vi "诊断标定4.vi"(8 "CAN端口":u16(ring), 9 "设备索引号":u16(ring), 10 "CAN卡类型":u32(ring)=4) -> ()   [LabVIEW 2013] (continued)
            n2064 = property on="SOH(%)" class="DigNum (严格)"("Disabled"=w3261) -> ()  [unwired: 2 in, 2 out]
            n2065 = property on="电池额定容量(A)" class="DigNum (严格)"("Disabled"=w3261) -> ()  [unwired: 2 in, 2 out]
            n2066 = property on="SOC(%)" class="DigNum (严格)"("Disabled"=w3261) -> ()  [unwired: 2 in, 2 out]
            n2067 = local read "从板个数"() -> (w3259:dbl)
            n2068 = property on="系统时钟" class="Str"("Disabled"=w3261) -> ()  [unwired: 2 in, 2 out]
            n2069 = property on="配置文件版本" class="Str"("Disabled"=w3261) -> ()  [unwired: 2 in, 2 out]
            n2070 = property on="车架(牌)号" class="Str"("Disabled"=w3261) -> ()  [unwired: 2 in, 2 out]
            n2071 = property on="产品编号" class="Str"("Disabled"=w3261) -> ()  [unwired: 2 in, 2 out]
            n2072 = control-ref of="项目信息"() -> (w3260:refnum<vi>)
            n2073 = stacked-sequence {
              tunnel: w3260 -> [w3272 w3275]
              tunnel: w3259 -> [w3265 w3274]
              frame #0 {
                n2074 = Multiply(x=w3265, y=4.0) -> (x*y=w3267:dbl)
                n2075 = Compound Arithmetic op=ADD(24.0 ("值"), w3267) -> (w3269:dbl)
                n2076 = Bundle(w3269, 0) -> (w3271:cluster{dbl, i32})  [unwired: 1 out]
                n2077 = property class="Tbl (严格)"(reference=w3272, "Index Values"=w3271) -> ()  [unwired: 1 in, 2 out]
              }
              frame #1 {
                n2078 = for {
                  N: 20 -> [_]
                  tunnel: w3275 -> [w3285]
                  tunnel: w3274 -> [w3280]
                  i -> [w3279]
                  n2079 = Multiply(x=4.0, y=w3280) -> (x*y=w3277:dbl)
                  n2080 = Compound Arithmetic op=ADD(24.0 ("值"), w3277, w3279) -> (w3282:dbl)
                  n2081 = Bundle(w3282, 0) -> (w3284:cluster{dbl, i32})  [unwired: 1 out]
                  n2082 = property class="Tbl (严格)"(reference=w3285, "Active Cell"=w3284, "Cell BG Color"=u32 6618880) -> ()  [unwired: 1 in, 2 out]
                }
              }
            }
            n2083 = Select(t=1, s=w3252, f=0) -> (s? t:f=w3250:i32)
            n2084 = global read "功能码全局.vi" "主板项目信息4"() -> (w3257:bool[])
            n2085 = property on="项目信息" class="Tbl (严格)"("Disabled"=w3250) -> ()  [unwired: 2 in, 2 out]
            n2086 = Index Array(array=w3257, index #1=5 ("索引"), index #2=6 ("索引")) -> (element #1=w3255:bool, element #2=w3254:bool)
            n2087 = Not(x=w3263) -> (.not. x?=w3262:bool)
          }
          frame "SOC" {
            w3295 = 2
            w3297 = FALSE
            n2088 = property on="电池实际容量(A)" class="DigNum (严格)"("Disabled"=w3295) -> ()  [unwired: 2 in, 2 out]
            n2089 = property on="使用者" class="DigNum (严格)"("Disabled"=w3295) -> ()  [unwired: 2 in, 2 out]
            n2090 = property on="SOH(%)" class="DigNum (严格)"("Disabled"=w3295) -> ()  [unwired: 2 in, 2 out]
            n2091 = property on="电池额定容量(A)" class="DigNum (严格)"("Disabled"=w3295) -> ()  [unwired: 2 in, 2 out]
            n2092 = property on="系统时钟" class="Str"("Disabled"=w3295) -> ()  [unwired: 2 in, 2 out]
            n2093 = property on="配置文件版本" class="Str"("Disabled"=w3295) -> ()  [unwired: 2 in, 2 out]
            n2094 = property on="车架(牌)号" class="Str"("Disabled"=w3295) -> ()  [unwired: 2 in, 2 out]
            n2095 = property on="项目信息" class="Tbl (严格)"("Disabled"=w3295) -> ()  [unwired: 2 in, 2 out]
            n2096 = property on="产品编号" class="Str"("Disabled"=w3295) -> ()  [unwired: 2 in, 2 out]
            n2097 = Select(t=0, s=w3287, f=1) -> (s? t:f=w3286:i32)
            n2098 = property on="SOC(%)" class="DigNum (严格)"("Disabled"=w3286) -> ()  [unwired: 2 in, 2 out]
            n2099 = global read "功能码全局.vi" "主板项目信息7"() -> (w3293:bool[])
            n2100 = Index Array(array=w3293, index #1=2 ("索引"), index #2=5 ("索引")) -> (element #1=w3291:bool, element #2=w3290:bool)
            n2101 = Not(x=w3297) -> (.not. x?=w3296:bool)
          }
          frame "电池额定实际容量" {
            w3308 = 2
            w3310 = FALSE
            n2102 = property on="使用者" class="DigNum (严格)"("Disabled"=w3308) -> ()  [unwired: 2 in, 2 out]
            n2103 = property on="SOH(%)" class="DigNum (严格)"("Disabled"=w3308) -> ()  [unwired: 2 in, 2 out]
            n2104 = property on="SOC(%)" class="DigNum (严格)"("Disabled"=w3308) -> ()  [unwired: 2 in, 2 out]
            n2105 = property on="系统时钟" class="Str"("Disabled"=w3308) -> ()  [unwired: 2 in, 2 out]
            n2106 = property on="配置文件版本" class="Str"("Disabled"=w3308) -> ()  [unwired: 2 in, 2 out]
            n2107 = property on="车架(牌)号" class="Str"("Disabled"=w3308) -> ()  [unwired: 2 in, 2 out]
            n2108 = property on="项目信息" class="Tbl (严格)"("Disabled"=w3308) -> ()  [unwired: 2 in, 2 out]
            n2109 = property on="产品编号" class="Str"("Disabled"=w3308) -> ()  [unwired: 2 in, 2 out]
            n2110 = Select(t=0, s=w3300, f=1) -> (s? t:f=w3299:i32)
            n2111 = property on="电池实际容量(A)" class="DigNum (严格)"("Disabled"=w3299) -> ()  [unwired: 2 in, 2 out]
            n2112 = property on="电池额定容量(A)" class="DigNum (严格)"("Disabled"=w3299) -> ()  [unwired: 2 in, 2 out]
            n2113 = global read "功能码全局.vi" "主板项目信息7"() -> (w3306:bool[])
            n2114 = Index Array(array=w3306, index #1=3 ("索引"), index #2=6 ("索引")) -> (element #1=w3304:bool, element #2=w3303:bool)
            n2115 = Not(x=w3310) -> (.not. x?=w3309:bool)
          }
          frame "配置文件版本" {
            w3322 = 2
            w3324 = FALSE
            n2116 = property on="使用者" class="DigNum (严格)"("Disabled"=w3322) -> ()  [unwired: 2 in, 2 out]
            n2117 = property on="SOH(%)" class="DigNum (严格)"("Disabled"=w3322) -> ()  [unwired: 2 in, 2 out]
            n2118 = property on="SOC(%)" class="DigNum (严格)"("Disabled"=w3322) -> ()  [unwired: 2 in, 2 out]
            n2119 = property on="电池实际容量(A)" class="DigNum (严格)"("Disabled"=w3322) -> ()  [unwired: 2 in, 2 out]
            n2120 = property on="电池额定容量(A)" class="DigNum (严格)"("Disabled"=w3322) -> ()  [unwired: 2 in, 2 out]
            n2121 = property on="系统时钟" class="Str"("Disabled"=w3322) -> ()  [unwired: 2 in, 2 out]
            n2122 = property on="车架(牌)号" class="Str"("Disabled"=w3322) -> ()  [unwired: 2 in, 2 out]
            n2123 = property on="项目信息" class="Tbl (严格)"("Disabled"=w3322) -> ()  [unwired: 2 in, 2 out]
            n2124 = property on="产品编号" class="Str"("Disabled"=w3322) -> ()  [unwired: 2 in, 2 out]
            n2125 = Select(t=0, s=w3313, f=1) -> (s? t:f=w3312:i32)
            n2126 = property on="配置文件版本" class="Str"("Disabled"=w3312) -> ()  [unwired: 2 in, 2 out]
            n2127 = global read "功能码全局.vi" "主板项目信息5"() -> (w3320:bool[])
            n2128 = global read "功能码全局.vi" "主板项目信息6"() -> (w3319:bool[])
            n2129 = Index Array(array=w3320, index=6 ("索引")) -> (element=w3317:bool)
            n2130 = Index Array(array=w3319, index=7 ("索引")) -> (element=w3316:bool)
            n2131 = Not(x=w3324) -> (.not. x?=w3323:bool)
          }
          frame "参数修改记录" {
            w3336 = 2
            w3338 = FALSE
            n2132 = property on="SOH(%)" class="DigNum (严格)"("Disabled"=w3336) -> ()  [unwired: 2 in, 2 out]
            n2133 = property on="SOC(%)" class="DigNum (严格)"("Disabled"=w3336) -> ()  [unwired: 2 in, 2 out]
            n2134 = property on="电池实际容量(A)" class="DigNum (严格)"("Disabled"=w3336) -> ()  [unwired: 2 in, 2 out]
            n2135 = property on="电池额定容量(A)" class="DigNum (严格)"("Disabled"=w3336) -> ()  [unwired: 2 in, 2 out]
            n2136 = property on="系统时钟" class="Str"("Disabled"=w3336) -> ()  [unwired: 2 in, 2 out]
            n2137 = property on="车架(牌)号" class="Str"("Disabled"=w3336) -> ()  [unwired: 2 in, 2 out]
            n2138 = property on="配置文件版本" class="Str"("Disabled"=w3336) -> ()  [unwired: 2 in, 2 out]
            n2139 = property on="项目信息" class="Tbl (严格)"("Disabled"=w3336) -> ()  [unwired: 2 in, 2 out]
            n2140 = property on="产品编号" class="Str"("Disabled"=w3336) -> ()  [unwired: 2 in, 2 out]
            n2141 = Select(t=0, s=w3327, f=1) -> (s? t:f=w3326:i32)
            n2142 = property on="使用者" class="DigNum (严格)"("Disabled"=w3326) -> ()  [unwired: 2 in, 2 out]
            n2143 = global read "功能码全局.vi" "主板项目信息7"() -> (w3333:bool[])
            n2144 = global read "功能码全局.vi" "主板项目信息5"() -> (w3334:bool[])
            n2145 = Index Array(array=w3333, index=0 ("索引")) -> (element=w3331:bool)
            n2146 = Index Array(array=w3334, index=7 ("索引")) -> (element=w3330:bool)
            n2147 = Not(x=w3338) -> (.not. x?=w3337:bool)
          }
          frame "车牌号" {
            w3350 = 2
            w3352 = FALSE
            n2148 = property on="SOH(%)" class="DigNum (严格)"("Disabled"=w3350) -> ()  [unwired: 2 in, 2 out]
            n2149 = property on="使用者" class="DigNum (严格)"("Disabled"=w3350) -> ()  [unwired: 2 in, 2 out]
            n2150 = property on="SOC(%)" class="DigNum (严格)"("Disabled"=w3350) -> ()  [unwired: 2 in, 2 out]
            n2151 = property on="电池实际容量(A)" class="DigNum (严格)"("Disabled"=w3350) -> ()  [unwired: 2 in, 2 out]
            n2152 = property on="电池额定容量(A)" class="DigNum (严格)"("Disabled"=w3350) -> ()  [unwired: 2 in, 2 out]
            n2153 = property on="系统时钟" class="Str"("Disabled"=w3350) -> ()  [unwired: 2 in, 2 out]
            n2154 = property on="配置文件版本" class="Str"("Disabled"=w3350) -> ()  [unwired: 2 in, 2 out]
            n2155 = property on="项目信息" class="Tbl (严格)"("Disabled"=w3350) -> ()  [unwired: 2 in, 2 out]
            n2156 = property on="产品编号" class="Str"("Disabled"=w3350) -> ()  [unwired: 2 in, 2 out]
            n2157 = Select(t=0, s=w3341, f=1) -> (s? t:f=w3340:i32)
            n2158 = property on="车架(牌)号" class="Str"("Disabled"=w3340) -> ()  [unwired: 2 in, 2 out]
            n2159 = global read "功能码全局.vi" "主板项目信息7"() -> (w3347:bool[])
            n2160 = global read "功能码全局.vi" "主板项目信息6"() -> (w3348:bool[])
            n2161 = Index Array(array=w3347, index=1 ("索引")) -> (element=w3345:bool)
            n2162 = Index Array(array=w3348, index=0 ("索引")) -> (element=w3344:bool)
            n2163 = Not(x=w3352) -> (.not. x?=w3351:bool)
          }
          frame "SOH" {
            w3363 = 2
            w3365 = FALSE
            n2164 = property on="使用者" class="DigNum (严格)"("Disabled"=w3363) -> ()  [unwired: 2 in, 2 out]
            n2165 = property on="SOC(%)" class="DigNum (严格)"("Disabled"=w3363) -> ()  [unwired: 2 in, 2 out]
            n2166 = property on="电池实际容量(A)" class="DigNum (严格)"("Disabled"=w3363) -> ()  [unwired: 2 in, 2 out]
            n2167 = property on="电池额定容量(A)" class="DigNum (严格)"("Disabled"=w3363) -> ()  [unwired: 2 in, 2 out]
            n2168 = property on="系统时钟" class="Str"("Disabled"=w3363) -> ()  [unwired: 2 in, 2 out]
            n2169 = property on="配置文件版本" class="Str"("Disabled"=w3363) -> ()  [unwired: 2 in, 2 out]
            n2170 = property on="项目信息" class="Tbl (严格)"("Disabled"=w3363) -> ()  [unwired: 2 in, 2 out]
            n2171 = property on="产品编号" class="Str"("Disabled"=w3363) -> ()  [unwired: 2 in, 2 out]
            n2172 = property on="车架(牌)号" class="Str"("Disabled"=w3363) -> ()  [unwired: 2 in, 2 out]
            n2173 = Select(t=0, s=w3355, f=1) -> (s? t:f=w3354:i32)
            n2174 = property on="SOH(%)" class="DigNum (严格)"("Disabled"=w3354) -> ()  [unwired: 2 in, 2 out]
            n2175 = global read "功能码全局.vi" "主板项目信息7"() -> (w3362:bool[])
            n2176 = Index Array(array=w3362, index #1=4 ("索引"), index #2=7 ("索引")) -> (element #1=w3359:bool, element #2=w3358:bool)
            n2177 = Not(x=w3365) -> (.not. x?=w3364:bool)
          }
          frame "SOC过低(2)", "SOC过高(2)", "SOH过低(2)", "充电电流过高(2)", "单体电压过低(2)", "单体电压过高(2)", "单组电压不均衡(2)", "单组温度不均衡(2)", "二级故障阀值", "放电电流过高(2)", "极柱温度过高(2)", "内阻过大(2)", "温度过低(2)", "温度过高(2)", "整组电压不均衡(2)", "整组温度不均衡(2)", "总电压过低(2)", "总电压过高(2)" {
            w3376 = FALSE
            n2178 = Select(t=0, s=w3368, f=1) -> (s? t:f=w3367:i32)
            n2179 = property on="一级故障 2" class="Clust (严格)"("DisabledEnum"=w3367) -> ()  [unwired: 2 in, 2 out]
            n2180 = global read "功能码全局.vi" "主板故障阀值9"() -> (w3374:bool[])
            n2181 = Index Array(array=w3374, index #1=3 ("索引"), index #2=6 ("索引")) -> (element #1=w3372:bool, element #2=w3371:bool)
            n2182 = Not(x=w3376) -> (.not. x?=w3377:bool)
          }
          frame "SOC过低(3)", "SOC过高(3)", "SOH过低(3)", "充电电流过高(3)", "单体电压过低(3)", "单体电压过高(3)", "单组电压不均衡(3)", "单组温度不均衡(3)", "放电电流过高(3)", "极柱温度过高(3)", "内阻过大(3)", "三级故障阀值", "温度过低(3)", "温度过高(3)", "整组电压不均衡(3)", "整组温度不均衡(3)", "总电压过低(3)", "总电压过高(3)" {
            w3389 = FALSE
            n2183 = Select(t=0, s=w3380, f=1) -> (s? t:f=w3379:i32)
            n2184 = property on="一级故障 3" class="Clust (严格)"("DisabledEnum"=w3379) -> ()  [unwired: 2 in, 2 out]
            n2185 = global read "功能码全局.vi" "主板故障阀值9"() -> (w3386:bool[])
            n2186 = Index Array(array=w3386, index #1=4 ("索引"), index #2=7 ("索引")) -> (element #1=w3384:bool, element #2=w3383:bool)
            n2187 = Not(x=w3389) -> (.not. x?=w3388:bool)
          }
          frame "SOC过低", "SOC过高", "SOH过低", "充电电流过高", "单体电压过低", "单体电压过高", "单组电压不均衡", "单组温度不均衡", "放电电流过高", "极柱温度过高", "内阻过大", "温度过低", "温度过高", "一级故障阀值", "整组电压不均衡", "整组温度不均衡", "总电压过低", "总电压过高" {
            w3401 = FALSE
            n2188 = Select(t=0, s=w3392, f=1) -> (s? t:f=w3391:i32)
            n2189 = property on="一级故障" class="Clust (严格)"("DisabledEnum"=w3391) -> ()  [unwired: 2 in, 2 out]
            n2190 = global read "功能码全局.vi" "主板故障阀值9"() -> (w3398:bool[])
            n2191 = Index Array(array=w3398, index #1=2 ("索引"), index #2=5 ("索引")) -> (element #1=w3396:bool, element #2=w3395:bool)
            n2192 = Not(x=w3401) -> (.not. x?=w3400:bool)
          }
          frame "充电控制参数", "电流步长", "最大允许充电电流", "最大允许充电温度", "最大允许单体电压", "最大允许总电压", "最小允许充电电流", "最小允许充电温度", "最小允许单体电压" {
            w3403 = 2
            w3414 = FALSE
            n2193 = property on="风机开启温度" class="DigNum (严格)"("Disabled"=w3403) -> ()  [unwired: 2 in, 2 out]
            n2194 = property on="风机关闭温度" class="DigNum (严格)"("Disabled"=w3403) -> ()  [unwired: 2 in, 2 out]
            n2195 = property on="加热开启温度" class="DigNum (严格)"("Disabled"=w3403) -> ()  [unwired: 2 in, 2 out]
            n2196 = property on="加热关闭温度" class="DigNum (严格)"("Disabled"=w3403) -> ()  [unwired: 2 in, 2 out]
            n2197 = property on="风机开启温差" class="DigNum (严格)"("Disabled"=w3403) -> ()  [unwired: 2 in, 2 out]
            n2198 = property on="风机关闭温差" class="DigNum (严格)"("Disabled"=w3403) -> ()  [unwired: 2 in, 2 out]
            n2199 = property on="加热控制参数" class="Clust (严格)"("DisabledEnum"=w3403) -> ()  [unwired: 2 in, 2 out]
            n2200 = Select(t=0, s=w3405, f=1) -> (s? t:f=w3404:i32)
            n2201 = property on="最大允许总电压" class="DigNum (严格)"("Disabled"=w3404) -> ()  [unwired: 2 in, 2 out]
            n2202 = property on="最大允许充电温度" class="DigNum (严格)"("Disabled"=w3404) -> ()  [unwired: 2 in, 2 out]
            n2203 = property on="最小允许充电温度" class="DigNum (严格)"("Disabled"=w3404) -> ()  [unwired: 2 in, 2 out]
            n2204 = property on="电流步长" class="DigNum (严格)"("Disabled"=w3404) -> ()  [unwired: 2 in, 2 out]
            n2205 = property on="最大允许单体电压" class="DigNum (严格)"("Disabled"=w3404) -> ()  [unwired: 2 in, 2 out]
            n2206 = property on="最小允许单体电压" class="DigNum (严格)"("Disabled"=w3404) -> ()  [unwired: 2 in, 2 out]
            n2207 = property on="最大允许充电电流" class="DigNum (严格)"("Disabled"=w3404) -> ()  [unwired: 2 in, 2 out]
            n2208 = property on="最小允许充电电流" class="DigNum (严格)"("Disabled"=w3404) -> ()  [unwired: 2 in, 2 out]
            n2209 = global read "功能码全局.vi" "主板控制类信息10"() -> (w3411:bool[])
            n2210 = Index Array(array=w3411, index #1=5 ("索引"), index #2=7 ("索引")) -> (element #1=w3409:bool, element #2=w3408:bool)
            n2211 = Not(x=w3414) -> (.not. x?=w3413:bool)
          }
          frame "风机关闭温差", "风机关闭温度", "风机开启温差", "风机开启温度", "加热关闭温差", "加热关闭温度", "加热开启温度", "加热控制参数" {
            w3425 = 2
            w3427 = FALSE
            n2212 = Select(t=0, s=w3417, f=1) -> (s? t:f=w3416:i32)
            n2213 = property on="加热控制参数" class="Clust (严格)"("DisabledEnum"=w3416) -> ()  [unwired: 2 in, 2 out]
            n2214 = property on="风机开启温度" class="DigNum (严格)"("Disabled"=w3416) -> ()  [unwired: 2 in, 2 out]
            n2215 = property on="风机关闭温度" class="DigNum (严格)"("Disabled"=w3416) -> ()  [unwired: 2 in, 2 out]
            n2216 = property on="加热开启温度" class="DigNum (严格)"("Disabled"=w3416) -> ()  [unwired: 2 in, 2 out]
            n2217 = property on="加热关闭温度" class="DigNum (严格)"("Disabled"=w3416) -> ()  [unwired: 2 in, 2 out]
            n2218 = property on="风机开启温差" class="DigNum (严格)"("Disabled"=w3416) -> ()  [unwired: 2 in, 2 out]
            n2219 = property on="风机关闭温差" class="DigNum (严格)"("Disabled"=w3416) -> ()  [unwired: 2 in, 2 out]
            n2220 = property on="最大允许总电压" class="DigNum (严格)"("Disabled"=w3425) -> ()  [unwired: 2 in, 2 out]
            n2221 = property on="最大允许充电温度" class="DigNum (严格)"("Disabled"=w3425) -> ()  [unwired: 2 in, 2 out]
            n2222 = property on="最小允许充电温度" class="DigNum (严格)"("Disabled"=w3425) -> ()  [unwired: 2 in, 2 out]
            n2223 = property on="电流步长" class="DigNum (严格)"("Disabled"=w3425) -> ()  [unwired: 2 in, 2 out]
            n2224 = property on="最大允许单体电压" class="DigNum (严格)"("Disabled"=w3425) -> ()  [unwired: 2 in, 2 out]
            n2225 = property on="最小允许单体电压" class="DigNum (严格)"("Disabled"=w3425) -> ()  [unwired: 2 in, 2 out]
            n2226 = property on="最大允许充电电流" class="DigNum (严格)"("Disabled"=w3425) -> ()  [unwired: 2 in, 2 out]
            n2227 = property on="最小允许充电电流" class="DigNum (严格)"("Disabled"=w3425) -> ()  [unwired: 2 in, 2 out]
            n2228 = global read "功能码全局.vi" "主板控制类信息10"() -> (w3423:bool[])
            n2229 = Index Array(array=w3423, index #1=4 ("索引"), index #2=6 ("索引")) -> (element #1=w3421:bool, element #2=w3420:bool)
            n2230 = Not(x=w3427) -> (.not. x?=w3426:bool)
          }
          frame "电池信息" {
            w3439 = FALSE
            n2231 = Select(t=0, s=w3430, f=1) -> (s? t:f=w3429:i32)
            n2232 = property on="电池串联" class="DigNum (严格)"("Disabled"=w3429) -> ()  [unwired: 2 in, 2 out]
            n2233 = property on="电池并联" class="DigNum (严格)"("Disabled"=w3429) -> ()  [unwired: 2 in, 2 out]
            n2234 = property on="电池包额定容量" class="DigNum (严格)"("Disabled"=w3429) -> ()  [unwired: 2 in, 2 out]
            n2235 = property on="电池包额定能量" class="DigNum (严格)"("Disabled"=w3429) -> ()  [unwired: 2 in, 2 out]
            n2236 = property on="电池包额定总电压" class="DigNum (严格)"("Disabled"=w3429) -> ()  [unwired: 2 in, 2 out]
            n2237 = property on="实际容量" class="DigNum (严格)"("Disabled"=w3429) -> ()  [unwired: 2 in, 2 out]
            n2238 = property on="电池包组号" class="Str"("Disabled"=w3429) -> ()  [unwired: 2 in, 2 out]
            n2239 = property on="电池生产日期" class="Str"("Disabled"=w3429) -> ()  [unwired: 2 in, 2 out]
            n2240 = property on="电池厂家" class="Str"("Disabled"=w3429) -> ()  [unwired: 2 in, 2 out]
            n2241 = property on="电池类型" class="Str"("Disabled"=w3429) -> ()  [unwired: 2 in, 2 out]
            n2242 = property on="累计充电总安时" class="DigNum (严格)"("Disabled"=w3429) -> ()  [unwired: 2 in, 2 out]
            n2243 = property on="累计放电总安时" class="DigNum (严格)"("Disabled"=w3429) -> ()  [unwired: 2 in, 2 out]
            n2244 = property on="电池放空次数" class="DigNum (严格)"("Disabled"=w3429) -> ()  [unwired: 2 in, 2 out]
            n2245 = property on="电池充满次数" class="DigNum (严格)"("Disabled"=w3429) -> ()  [unwired: 2 in, 2 out]
            n2246 = property on="电池充电次数" class="DigNum (严格)"("Disabled"=w3429) -> ()  [unwired: 2 in, 2 out]
            n2247 = global read "功能码全局.vi" "主板版本号11"() -> (w3436:bool[])
            n2248 = Index Array(array=w3436, index #1=0 ("索引"), index #2=1 ("索引")) -> (element #1=w3434:bool, element #2=w3433:bool)
            n2249 = Not(x=w3439) -> (.not. x?=w3438:bool)
          }
          frame "电池信息1" {
            w3450 = 2
            w3452 = FALSE
            n2250 = Select(t=0, s=w3441, f=1) -> (s? t:f=w3442:i32)
            n2251 = property on="电池生产日期" class="Str"("Disabled"=w3442) -> ()  [unwired: 2 in, 2 out]
            n2252 = property on="电池厂家" class="Str"("Disabled"=w3442) -> ()  [unwired: 2 in, 2 out]
            n2253 = property on="电池类型" class="Str"("Disabled"=w3442) -> ()  [unwired: 2 in, 2 out]
            n2254 = property on="电池串联" class="DigNum (严格)"("Disabled"=w3442) -> ()  [unwired: 2 in, 2 out]
            n2255 = property on="电池并联" class="DigNum (严格)"("Disabled"=w3442) -> ()  [unwired: 2 in, 2 out]
            n2256 = property on="电池包额定容量" class="DigNum (严格)"("Disabled"=w3442) -> ()  [unwired: 2 in, 2 out]
            n2257 = property on="电池包额定能量" class="DigNum (严格)"("Disabled"=w3442) -> ()  [unwired: 2 in, 2 out]
            n2258 = property on="电池包额定总电压" class="DigNum (严格)"("Disabled"=w3442) -> ()  [unwired: 2 in, 2 out]
            n2259 = property on="实际容量" class="DigNum (严格)"("Disabled"=w3442) -> ()  [unwired: 2 in, 2 out]
            n2260 = property on="累计充电总安时" class="DigNum (严格)"("Disabled"=w3450) -> ()  [unwired: 2 in, 2 out]
            n2261 = property on="累计放电总安时" class="DigNum (严格)"("Disabled"=w3450) -> ()  [unwired: 2 in, 2 out]
            n2262 = property on="电池放空次数" class="DigNum (严格)"("Disabled"=w3450) -> ()  [unwired: 2 in, 2 out]
            n2263 = property on="电池充满次数" class="DigNum (严格)"("Disabled"=w3450) -> ()  [unwired: 2 in, 2 out]
            n2264 = property on="电池充电次数" class="DigNum (严格)"("Disabled"=w3450) -> ()  [unwired: 2 in, 2 out]
            n2265 = property on="电池包组号" class="Str"("Disabled"=w3450) -> ()  [unwired: 2 in, 2 out]
            n2266 = global read "功能码全局.vi" "主板版本号11"() -> (w3448:bool[])
            n2267 = Index Array(array=w3448, index #1=0 ("索引"), index #2=1 ("索引")) -> (element #1=w3446:bool, element #2=w3445:bool)
            n2268 = Not(x=w3452) -> (.not. x?=w3451:bool)
          }
          frame "电池包组号" {
            w3463 = 2
            w3465 = FALSE
            n2269 = property on="电池生产日期" class="Str"("Disabled"=w3463) -> ()  [unwired: 2 in, 2 out]
            n2270 = property on="电池厂家" class="Str"("Disabled"=w3463) -> ()  [unwired: 2 in, 2 out]
            n2271 = property on="电池类型" class="Str"("Disabled"=w3463) -> ()  [unwired: 2 in, 2 out]
            n2272 = property on="电池串联" class="DigNum (严格)"("Disabled"=w3463) -> ()  [unwired: 2 in, 2 out]
            n2273 = property on="电池并联" class="DigNum (严格)"("Disabled"=w3463) -> ()  [unwired: 2 in, 2 out]
            n2274 = property on="电池包额定容量" class="DigNum (严格)"("Disabled"=w3463) -> ()  [unwired: 2 in, 2 out]
            n2275 = property on="电池包额定能量" class="DigNum (严格)"("Disabled"=w3463) -> ()  [unwired: 2 in, 2 out]
            n2276 = property on="电池包额定总电压" class="DigNum (严格)"("Disabled"=w3463) -> ()  [unwired: 2 in, 2 out]
            n2277 = property on="实际容量" class="DigNum (严格)"("Disabled"=w3463) -> ()  [unwired: 2 in, 2 out]
            n2278 = property on="累计充电总安时" class="DigNum (严格)"("Disabled"=w3463) -> ()  [unwired: 2 in, 2 out]
            n2279 = property on="累计放电总安时" class="DigNum (严格)"("Disabled"=w3463) -> ()  [unwired: 2 in, 2 out]
            n2280 = property on="电池放空次数" class="DigNum (严格)"("Disabled"=w3463) -> ()  [unwired: 2 in, 2 out]
            n2281 = property on="电池充满次数" class="DigNum (严格)"("Disabled"=w3463) -> ()  [unwired: 2 in, 2 out]
            n2282 = property on="电池充电次数" class="DigNum (严格)"("Disabled"=w3463) -> ()  [unwired: 2 in, 2 out]
            n2283 = Select(t=0, s=w3455, f=1) -> (s? t:f=w3454:i32)
            n2284 = property on="电池包组号" class="Str"("Disabled"=w3454) -> ()  [unwired: 2 in, 2 out]
            n2285 = global read "功能码全局.vi" "主板版本号11"() -> (w3461:bool[])
            n2286 = Index Array(array=w3461, index #1=0 ("索引"), index #2=1 ("索引")) -> (element #1=w3459:bool, element #2=w3458:bool)
            n2287 = Not(x=w3465) -> (.not. x?=w3464:bool)
          }
          frame "充放电安时" {
            w3476 = 2
            w3478 = FALSE
            n2288 = property on="电池生产日期" class="Str"("Disabled"=w3476) -> ()  [unwired: 2 in, 2 out]
            n2289 = property on="电池厂家" class="Str"("Disabled"=w3476) -> ()  [unwired: 2 in, 2 out]
            n2290 = property on="电池类型" class="Str"("Disabled"=w3476) -> ()  [unwired: 2 in, 2 out]
            n2291 = property on="电池串联" class="DigNum (严格)"("Disabled"=w3476) -> ()  [unwired: 2 in, 2 out]
            n2292 = property on="电池并联" class="DigNum (严格)"("Disabled"=w3476) -> ()  [unwired: 2 in, 2 out]
            n2293 = property on="电池包额定容量" class="DigNum (严格)"("Disabled"=w3476) -> ()  [unwired: 2 in, 2 out]
            n2294 = property on="电池包额定能量" class="DigNum (严格)"("Disabled"=w3476) -> ()  [unwired: 2 in, 2 out]
            n2295 = property on="电池包额定总电压" class="DigNum (严格)"("Disabled"=w3476) -> ()  [unwired: 2 in, 2 out]
            n2296 = property on="实际容量" class="DigNum (严格)"("Disabled"=w3476) -> ()  [unwired: 2 in, 2 out]
            n2297 = property on="电池放空次数" class="DigNum (严格)"("Disabled"=w3476) -> ()  [unwired: 2 in, 2 out]
            n2298 = property on="电池充满次数" class="DigNum (严格)"("Disabled"=w3476) -> ()  [unwired: 2 in, 2 out]
            n2299 = property on="电池充电次数" class="DigNum (严格)"("Disabled"=w3476) -> ()  [unwired: 2 in, 2 out]
            n2300 = Select(t=0, s=w3468, f=1) -> (s? t:f=w3467:i32)
            n2301 = property on="电池包组号" class="Str"("Disabled"=w3476) -> ()  [unwired: 2 in, 2 out]
            n2302 = property on="累计充电总安时" class="DigNum (严格)"("Disabled"=w3467) -> ()  [unwired: 2 in, 2 out]
            n2303 = property on="累计放电总安时" class="DigNum (严格)"("Disabled"=w3467) -> ()  [unwired: 2 in, 2 out]
            n2304 = global read "功能码全局.vi" "主板版本号11"() -> (w3474:bool[])
            n2305 = Index Array(array=w3474, index #1=0 ("索引"), index #2=1 ("索引")) -> (element #1=w3472:bool, element #2=w3471:bool)
            n2306 = Not(x=w3478) -> (.not. x?=w3477:bool)
          }
          frame "电池充放电次数" {
            w3489 = 2
            w3491 = FALSE
            n2307 = property on="电池生产日期" class="Str"("Disabled"=w3489) -> ()  [unwired: 2 in, 2 out]
            n2308 = property on="电池厂家" class="Str"("Disabled"=w3489) -> ()  [unwired: 2 in, 2 out]
            n2309 = property on="电池类型" class="Str"("Disabled"=w3489) -> ()  [unwired: 2 in, 2 out]
            n2310 = property on="电池串联" class="DigNum (严格)"("Disabled"=w3489) -> ()  [unwired: 2 in, 2 out]
            n2311 = property on="电池并联" class="DigNum (严格)"("Disabled"=w3489) -> ()  [unwired: 2 in, 2 out]
            n2312 = property on="电池包额定容量" class="DigNum (严格)"("Disabled"=w3489) -> ()  [unwired: 2 in, 2 out]
            n2313 = property on="电池包额定能量" class="DigNum (严格)"("Disabled"=w3489) -> ()  [unwired: 2 in, 2 out]
            n2314 = property on="电池包额定总电压" class="DigNum (严格)"("Disabled"=w3489) -> ()  [unwired: 2 in, 2 out]
            n2315 = property on="实际容量" class="DigNum (严格)"("Disabled"=w3489) -> ()  [unwired: 2 in, 2 out]
            n2316 = Select(t=0, s=w3481, f=1) -> (s? t:f=w3480:i32)
            n2317 = property on="电池放空次数" class="DigNum (严格)"("Disabled"=w3480) -> ()  [unwired: 2 in, 2 out]
            n2318 = property on="电池充满次数" class="DigNum (严格)"("Disabled"=w3480) -> ()  [unwired: 2 in, 2 out]
            n2319 = property on="电池充电次数" class="DigNum (严格)"("Disabled"=w3480) -> ()  [unwired: 2 in, 2 out]
            n2320 = property on="累计充电总安时" class="DigNum (严格)"("Disabled"=w3489) -> ()  [unwired: 2 in, 2 out]
            n2321 = property on="累计放电总安时" class="DigNum (严格)"("Disabled"=w3489) -> ()  [unwired: 2 in, 2 out]
            n2322 = property on="电池包组号" class="Str"("Disabled"=w3489) -> ()  [unwired: 2 in, 2 out]
            n2323 = global read "功能码全局.vi" "主板版本号11"() -> (w3487:bool[])
            n2324 = Index Array(array=w3487, index #1=0 ("索引"), index #2=1 ("索引")) -> (element #1=w3485:bool, element #2=w3484:bool)
            n2325 = Not(x=w3491) -> (.not. x?=w3490:bool)
          }
          frame "假", Default {
            w3496 = FALSE
            n2326 = Not(x=w3496) -> (.not. x?=w3495:bool)
          }
        }
        n2327 = property on="单个读取" class="Bool (严格)"("Visible"=w2991) -> ()  [unwired: 2 in, 2 out]
        n2328 = property on="单个写入" class="Bool (严格)"("Visible"=w2990) -> ()  [unwired: 2 in, 2 out]
        n2329 = local write "1"(w2998) -> ()
        n2330 = local write "1 2"(w2997) -> ()
        n2331 = local write "1 3"(w2996) -> ()
        n2332 = local write "1 4"(w2995) -> ()
        n2333 = local write "1 5"(w2994) -> ()
        n2334 = local write "1 11"(w2993) -> ()
        n2335 = local write "主板2"(w2999) -> ()
      }
      event "从板选项": Mouse Down {
        n2336 = event-data() -> ("CtlRef"=w3507:refnum<vi>)  [unwired: 8 out]
        n2337 = property class="Tree (严格)"(reference=w3507) -> ("Value"=w3506:string)  [unwired: 1 in, 2 out]
        n2338 = case shown="\"SOC过低(3)\", \"电压不均衡(3)\", \"电压过低(3)\", \"电压过高(3)\", \"三级故障阀值\", \"温度不均衡(3)\", \"温度过低(3)\", \"温度过高(3)\"" w3506 {
          tunnel: [T13."从板信息" ("等级 2") T13."从板信息" ("等级 2") T13."从板信息" ("等级 2") T13."从板信息" ("等级 2") T13."从板信息" ("等级 2") T13."从板信息" ("等级 2") T13."从板信息" ("等级 2") T13."一级故障阀值" ("等级 2") T13."二级故障阀值" ("等级 2") T13."三级故障阀值" ("等级 2") T13."快换参数" ("等级 2") T13."快换参数" ("等级 2") T13."快换参数" ("等级 2") T13."快换参数" ("等级 2") T13."快换参数" ("等级 2") T13."快换参数" ("等级 2") T13."快换参数" ("等级 2") T13."快换参数" ("等级 2") T13."从板信息" ("等级 2")] -> w3505
          tunnel: [w3516 w3521 w3531 w3542 w3573 w3606 w3630 w3661 w3669 w3677 w3682 w3691 w3700 w3710 w3720 w3731 w3742 w3752 w3754] -> w3504
          tunnel: [w3517 w3522 w3532 w3543 w3574 w3607 w3631 w3660 w3669 w3677 w3682 w3691 w3700 w3710 w3720 w3731 w3742 w3752 w3755] -> w3503
          tunnel: [w3517 w3522 w3532 w3543 w3574 w3607 w3631 w3661 w3668 w3677 w3682 w3691 w3700 w3710 w3720 w3731 w3742 w3752 w3755] -> w3502
          tunnel: [w3517 w3522 w3532 w3543 w3574 w3607 w3631 w3661 w3669 w3676 w3682 w3691 w3700 w3710 w3720 w3731 w3742 w3752 w3755] -> w3501
          tunnel: [w3517 w3522 w3532 w3543 w3574 w3607 w3631 w3661 w3669 w3677 w3681 w3690 w3699 w3709 w3719 w3730 w3741 w3751 w3755] -> w3500
          tunnel: [w3513 w3519 w3525 w3535 w3566 w3599 w3623 w3656 w3664 w3672 FALSE _ _ _ _ _ _ _ _] -> w3499
          tunnel: [w3510 w3519 w3524 w3534 w3565 w3598 w3622 w3655 w3663 w3671 _ _ _ _ _ _ _ _ _] -> w3498
          frame "从板号" {
            w3515 = 2
            w3517 = FALSE ("1 6")
            n2339 = property on="项目信息 2" class="Tbl (严格)"("Disabled"=w3515) -> ()  [unwired: 2 in, 2 out]
            n2340 = property on="加热控制参数" class="Clust (严格)"("Disabled"=w3515) -> ()  [unwired: 2 in, 2 out]
            n2341 = global read "功能码全局.vi" "16"() -> (w3512:bool[])
            n2342 = Index Array(array=w3512, index #1=4 ("索引"), index #2=6 ("索引")) -> (element #1=w3513:bool, element #2=w3510:bool)
            n2343 = Not(x=w3517) -> (.not. x?=w3516:bool)
          }
          frame "从板信息" {
            w3519 = TRUE
            w3520 = 0
            w3522 = FALSE ("1 6")
            n2344 = property on="项目信息 2" class="Tbl (严格)"("Disabled"=w3520) -> ()  [unwired: 2 in, 2 out]
            n2345 = property on="加热控制参数" class="Clust (严格)"("Disabled"=w3520) -> ()  [unwired: 2 in, 2 out]
            n2346 = Not(x=w3522) -> (.not. x?=w3521:bool)
          }
          frame "风机关闭温差", "风机关闭温度", "风机开启温差", "风机开启温度", "加热关闭温差", "加热关闭温度", "加热开启温度", "加热控制参数" {
            w3532 = FALSE ("1 6")
            n2347 = property on="项目信息 2" class="Tbl (严格)"("Disabled"=2) -> ()  [unwired: 2 in, 2 out]
            n2348 = property on="加热控制参数" class="Clust (严格)"("Disabled"=0) -> ()  [unwired: 2 in, 2 out]
            n2349 = global read "功能码全局.vi" "16"() -> (w3527:bool[])
            n2350 = Index Array(array=w3527, index #1=5 ("索引"), index #2=7 ("索引")) -> (element #1=w3525:bool, element #2=w3524:bool)
            n2351 = Not(x=w3532) -> (.not. x?=w3531:bool)
          }
          frame "电压起始值" {
            w3543 = FALSE ("1 6")
            n2352 = property on="项目信息 2" class="Tbl (严格)"("Disabled"=0) -> ()  [unwired: 2 in, 2 out]
            n2353 = property on="加热控制参数" class="Clust (严格)"("Disabled"=2) -> ()  [unwired: 2 in, 2 out]
            n2354 = control-ref of="项目信息 2"() -> (w3539:refnum<vi>)
            n2355 = stacked-sequence {
              tunnel: w3539 -> [w3548 w3550 w3559]
              frame #0 {
                n2356 = Bundle(0, 0) -> (w3547:cluster{i32, i32})  [unwired: 1 out]
                n2357 = property class="Tbl (严格)"(reference=w3548, "Index Values"=w3547) -> ()  [unwired: 1 in, 2 out]
              }
              frame #1 {
                n2358 = for {
                  N: 8 -> [_]
                  tunnel: w3550 -> [w3557]
                  i -> [w3552]
                  n2359 = Compound Arithmetic op=ADD(2 ("值"), w3552) -> (w3554:i32)
                  n2360 = Bundle(w3554, 0) -> (w3556:cluster{i32, i32})  [unwired: 1 out]
                  n2361 = property class="Tbl (严格)"(reference=w3557, "Active Cell"=w3556, "Cell BG Color"=u32 16448250) -> ()  [unwired: 1 in, 2 out]
                }
              }
              frame #2 {
                n2362 = for {
                  N: 2 -> [_]
                  tunnel: w3559 -> [w3564]
                  i -> [w3560]
                  n2363 = Bundle(w3560, 0) -> (w3563:cluster{i32, i32})  [unwired: 1 out]
                  n2364 = property class="Tbl (严格)"(reference=w3564, "Active Cell"=w3563, "Cell BG Color"=u32 6618880) -> ()  [unwired: 1 in, 2 out]
                }
              }
            }
            n2365 = global read "功能码全局.vi" "15"() -> (w3537:bool[])
            n2366 = Index Array(array=w3537, index #1=0 ("索引"), index #2=4 ("索引")) -> (element #1=w3535:bool, element #2=w3534:bool)
            n2367 = Not(x=w3543) -> (.not. x?=w3542:bool)
          }
          frame "通道电压节数" {
            w3574 = FALSE ("1 6")
            n2368 = property on="项目信息 2" class="Tbl (严格)"("Disabled"=0) -> ()  [unwired: 2 in, 2 out]
            n2369 = property on="加热控制参数" class="Clust (严格)"("Disabled"=2) -> ()  [unwired: 2 in, 2 out]
            n2370 = control-ref of="项目信息 2"() -> (w3570:refnum<vi>)
            n2371 = stacked-sequence {
              tunnel: w3570 -> [w3579 w3581 w3590]
              frame #0 {
                n2372 = Bundle(2, 0) -> (w3578:cluster{i32, i32})  [unwired: 1 out]
                n2373 = property class="Tbl (严格)"(reference=w3579, "Index Values"=w3578) -> ()  [unwired: 1 in, 2 out]
              }
              frame #1 {
                n2374 = for {
                  N: 8 -> [_]
                  tunnel: w3581 -> [w3588]
                  i -> [w3583]
                  n2375 = Compound Arithmetic op=ADD(12 ("值"), w3583) -> (w3585:i32)
                  n2376 = Bundle(w3585, 0) -> (w3587:cluster{i32, i32})  [unwired: 1 out]
                  n2377 = property class="Tbl (严格)"(reference=w3588, "Active Cell"=w3587, "Cell BG Color"=u32 16448250) -> ()  [unwired: 1 in, 2 out]
                }
              }
              frame #2 {
                n2378 = for {
                  N: 20 -> [_]
                  tunnel: w3590 -> [w3597]
                  i -> [w3593]
                  n2379 = Add(x=2, y=w3593) -> (x+y=w3592:i32)
                  n2380 = Bundle(w3592, 0) -> (w3596:cluster{i32, i32})  [unwired: 1 out]
                  n2381 = property class="Tbl (严格)"(reference=w3597, "Active Cell"=w3596, "Cell BG Color"=u32 6618880) -> ()  [unwired: 1 in, 2 out]
                }
              }
            }
            n2382 = global read "功能码全局.vi" "15"() -> (w3568:bool[])
            n2383 = Index Array(array=w3568, index #1=1 ("索引"), index #2=5 ("索引")) -> (element #1=w3566:bool, element #2=w3565:bool)
            n2384 = Not(x=w3574) -> (.not. x?=w3573:bool)
          }
          frame "保险位置" {
            w3607 = FALSE ("1 6")
            n2385 = property on="项目信息 2" class="Tbl (严格)"("Disabled"=0) -> ()  [unwired: 2 in, 2 out]
            n2386 = property on="加热控制参数" class="Clust (严格)"("Disabled"=2) -> ()  [unwired: 2 in, 2 out]
            n2387 = control-ref of="项目信息 2"() -> (w3603:refnum<vi>)
            n2388 = stacked-sequence {
              tunnel: w3603 -> [w3612 w3614]
              frame #0 {
                n2389 = Bundle(24, 0) -> (w3611:cluster{i32, i32})  [unwired: 1 out]
                n2390 = property class="Tbl (严格)"(reference=w3612, "Index Values"=w3611) -> ()  [unwired: 1 in, 2 out]
              }
              frame #1 {
                n2391 = for {
                  N: 20 -> [_]
                  tunnel: w3614 -> [w3621]
                  i -> [w3617]
                  n2392 = Add(x=24, y=w3617) -> (x+y=w3616:i32)
                  n2393 = Bundle(w3616, 0) -> (w3620:cluster{i32, i32})  [unwired: 1 out]
                  n2394 = property class="Tbl (严格)"(reference=w3621, "Active Cell"=w3620, "Cell BG Color"=u32 6618880) -> ()  [unwired: 1 in, 2 out]
                }
              }
            }
            n2395 = global read "功能码全局.vi" "15"() -> (w3601:bool[])
            n2396 = Index Array(array=w3601, index #1=2 ("索引"), index #2=6 ("索引")) -> (element #1=w3599:bool, element #2=w3598:bool)
            n2397 = Not(x=w3607) -> (.not. x?=w3606:bool)
          }
          frame "温度起始值" {
            w3631 = FALSE ("1 6")
            n2398 = property on="项目信息 2" class="Tbl (严格)"("Disabled"=0) -> ()  [unwired: 2 in, 2 out]
            n2399 = property on="加热控制参数" class="Clust (严格)"("Disabled"=2) -> ()  [unwired: 2 in, 2 out]
            n2400 = control-ref of="项目信息 2"() -> (w3627:refnum<vi>)
            n2401 = stacked-sequence {
              tunnel: w3627 -> [w3636 w3637 w3647]
              frame #0 {
                n2402 = Bundle(22, 0) -> (w3635:cluster{i32, i32})  [unwired: 1 out]
                n2403 = property class="Tbl (严格)"(reference=w3636, "Index Values"=w3635) -> ()  [unwired: 1 in, 2 out]
              }
              frame #1 {
                n2404 = for {
                  N: 10 -> [_]
                  tunnel: w3637 -> [w3645]
                  i -> [w3640]
                  n2405 = Compound Arithmetic op=ADD(24 ("值"), w3640) -> (w3642:i32)
                  n2406 = Bundle(w3642, 0) -> (w3644:cluster{i32, i32})  [unwired: 1 out]
                  n2407 = property class="Tbl (严格)"(reference=w3645, "Active Cell"=w3644, "Cell BG Color"=u32 16448250) -> ()  [unwired: 1 in, 2 out]
                }
              }
              frame #2 {
                n2408 = for {
                  N: 2 -> [_]
                  tunnel: w3647 -> [w3654]
                  i -> [w3650]
                  n2409 = Add(x=22, y=w3650) -> (x+y=w3649:i32)
                  n2410 = Bundle(w3649, 0) -> (w3653:cluster{i32, i32})  [unwired: 1 out]
                  n2411 = property class="Tbl (严格)"(reference=w3654, "Active Cell"=w3653, "Cell BG Color"=u32 6618880) -> ()  [unwired: 1 in, 2 out]
                }
              }
            }
            n2412 = global read "功能码全局.vi" "15"() -> (w3625:bool[])
            n2413 = Index Array(array=w3625, index #1=3 ("索引"), index #2=7 ("索引")) -> (element #1=w3623:bool, element #2=w3622:bool)
            n2414 = Not(x=w3631) -> (.not. x?=w3630:bool)
          }
          frame "SOC过低", "电压不均衡", "电压过低", "电压过高", "温度不均衡", "温度过低", "温度过高", "一级故障阀值" {
            w3661 = FALSE ("1 6")
            n2415 = global read "功能码全局.vi" "18"() -> (w3658:bool[])
            n2416 = Index Array(array=w3658, index #1=2 ("索引"), index #2=5 ("索引")) -> (element #1=w3656:bool, element #2=w3655:bool)
            n2417 = Not(x=w3661) -> (.not. x?=w3660:bool)
          }
          frame "SOC过低(2)", "电压不均衡(2)", "电压过低(2)", "电压过高(2)", "二级故障阀值", "温度不均衡(2)", "温度过低(2)", "温度过高(2)" {
            w3669 = FALSE ("1 6")
            n2418 = global read "功能码全局.vi" "18"() -> (w3666:bool[])
            n2419 = Index Array(array=w3666, index #1=3 ("索引"), index #2=6 ("索引")) -> (element #1=w3664:bool, element #2=w3663:bool)
            n2420 = Not(x=w3669) -> (.not. x?=w3668:bool)
          }
          frame "SOC过低(3)", "电压不均衡(3)", "电压过低(3)", "电压过高(3)", "三级故障阀值", "温度不均衡(3)", "温度过低(3)", "温度过高(3)" {
            w3677 = FALSE ("1 6")
            n2421 = global read "功能码全局.vi" "18"() -> (w3674:bool[])
            n2422 = Index Array(array=w3674, index #1=4 ("索引"), index #2=7 ("索引")) -> (element #1=w3672:bool, element #2=w3671:bool)
            n2423 = Not(x=w3677) -> (.not. x?=w3676:bool)
          }
          frame "快换参数" {
            w3682 = FALSE ("1 6")
            n2424 = property on="电池组信息" class="Clust (严格)"("Disabled"=0) -> ()  [unwired: 2 in, 2 out]
            n2425 = Not(x=w3682) -> (.not. x?=w3681:bool)
          }
          frame "电池包信息1" {
            w3684 = 2
            w3686 = 2
            w3688 = 0
            w3691 = FALSE ("1 6")
            n2426 = property on="电池类型" class="DigNum (严格)"("Disabled"=w3688) -> ()  [unwired: 2 in, 2 out]
            n2427 = property on="电池厂家" class="DigNum (严格)"("Disabled"=w3688) -> ()  [unwired: 2 in, 2 out]
            n2428 = property on="电池地区" class="DigNum (严格)"("Disabled"=w3688) -> ()  [unwired: 2 in, 2 out]
            n2429 = property on="电池组序号" class="DigNum (严格)"("Disabled"=w3688) -> ()  [unwired: 2 in, 2 out]
            n2430 = property on="电池包串联数" class="DigNum (严格)"("Disabled"=w3688) -> ()  [unwired: 2 in, 2 out]
            n2431 = property on="电池包并联数" class="DigNum (严格)"("Disabled"=w3688) -> ()  [unwired: 2 in, 2 out]
            n2432 = property on="电池包安时数" class="DigNum (严格)"("Disabled"=w3688) -> ()  [unwired: 2 in, 2 out]
            n2433 = property on="电池组信息" class="Clust (严格)"("Disabled"=0) -> ()  [unwired: 2 in, 2 out]
            n2434 = property on="车牌号" class="Str"("Disabled"=2) -> ()  [unwired: 2 in, 2 out]
            n2435 = property on="电池包序号" class="DigNum (严格)"("Disabled"=2) -> ()  [unwired: 2 in, 2 out]
            n2436 = property on="充电次数" class="DigNum (严格)"("Disabled"=w3686) -> ()  [unwired: 2 in, 2 out]
            n2437 = property on="充满电时间" class="DigNum (严格)"("Disabled"=w3686) -> ()  [unwired: 2 in, 2 out]
            n2438 = property on="放空时间" class="DigNum (严格)"("Disabled"=w3686) -> ()  [unwired: 2 in, 2 out]
            n2439 = property on="最大允许单体电压" class="DigNum (严格)"("Disabled"=w3684) -> ()  [unwired: 2 in, 2 out]
            n2440 = property on="最大允许总电压" class="DigNum (严格)"("Disabled"=w3684) -> ()  [unwired: 2 in, 2 out]
            n2441 = property on="最大允许温度" class="DigNum (严格)"("Disabled"=w3684) -> ()  [unwired: 2 in, 2 out]
            n2442 = property on="最小允许温度" class="DigNum (严格)"("Disabled"=w3684) -> ()  [unwired: 2 in, 2 out]
            n2443 = property on="最大允许充电电流" class="DigNum (严格)"("Disabled"=w3684) -> ()  [unwired: 2 in, 2 out]
            n2444 = property on="最小允许充电电流" class="DigNum (严格)"("Disabled"=w3684) -> ()  [unwired: 2 in, 2 out]
            n2445 = property on="最小允许单体电压" class="DigNum (严格)"("Disabled"=w3684) -> ()  [unwired: 2 in, 2 out]
            n2446 = property on="电流步长" class="DigNum (严格)"("Disabled"=w3684) -> ()  [unwired: 2 in, 2 out]
            n2447 = property on="SOC" class="DigNum (严格)"("Disabled"=w3684) -> ()  [unwired: 2 in, 2 out]
            n2448 = property on="充电总安时" class="DigNum (严格)"("Disabled"=w3684) -> ()  [unwired: 2 in, 2 out]
            n2449 = property on="放电总这时" class="DigNum (严格)"("Disabled"=w3684) -> ()  [unwired: 2 in, 2 out]
            n2450 = Not(x=w3691) -> (.not. x?=w3690:bool)
          }
          frame "电池包序号" {
            w3693 = 2
            w3695 = 2
            w3697 = 2
            w3700 = FALSE ("1 6")
            n2451 = property on="电池类型" class="DigNum (严格)"("Disabled"=w3697) -> ()  [unwired: 2 in, 2 out]
            n2452 = property on="电池厂家" class="DigNum (严格)"("Disabled"=w3697) -> ()  [unwired: 2 in, 2 out]
            n2453 = property on="电池地区" class="DigNum (严格)"("Disabled"=w3697) -> ()  [unwired: 2 in, 2 out]
            n2454 = property on="电池组序号" class="DigNum (严格)"("Disabled"=w3697) -> ()  [unwired: 2 in, 2 out]
            n2455 = property on="电池包串联数" class="DigNum (严格)"("Disabled"=w3697) -> ()  [unwired: 2 in, 2 out]
            n2456 = property on="电池包并联数" class="DigNum (严格)"("Disabled"=w3697) -> ()  [unwired: 2 in, 2 out]
            n2457 = property on="电池包安时数" class="DigNum (严格)"("Disabled"=w3697) -> ()  [unwired: 2 in, 2 out]
            n2458 = property on="电池组信息" class="Clust (严格)"("Disabled"=0) -> ()  [unwired: 2 in, 2 out]
            n2459 = property on="车牌号" class="Str"("Disabled"=2) -> ()  [unwired: 2 in, 2 out]
            n2460 = property on="电池包序号" class="DigNum (严格)"("Disabled"=0) -> ()  [unwired: 2 in, 2 out]
            n2461 = property on="充电次数" class="DigNum (严格)"("Disabled"=w3695) -> ()  [unwired: 2 in, 2 out]
            n2462 = property on="充满电时间" class="DigNum (严格)"("Disabled"=w3695) -> ()  [unwired: 2 in, 2 out]
            n2463 = property on="放空时间" class="DigNum (严格)"("Disabled"=w3695) -> ()  [unwired: 2 in, 2 out]
            n2464 = property on="最大允许单体电压" class="DigNum (严格)"("Disabled"=w3693) -> ()  [unwired: 2 in, 2 out]
            n2465 = property on="最大允许总电压" class="DigNum (严格)"("Disabled"=w3693) -> ()  [unwired: 2 in, 2 out]
            n2466 = property on="最大允许温度" class="DigNum (严格)"("Disabled"=w3693) -> ()  [unwired: 2 in, 2 out]
            n2467 = property on="最小允许温度" class="DigNum (严格)"("Disabled"=w3693) -> ()  [unwired: 2 in, 2 out]
            n2468 = property on="最大允许充电电流" class="DigNum (严格)"("Disabled"=w3693) -> ()  [unwired: 2 in, 2 out]
            n2469 = property on="最小允许充电电流" class="DigNum (严格)"("Disabled"=w3693) -> ()  [unwired: 2 in, 2 out]
            n2470 = property on="最小允许单体电压" class="DigNum (严格)"("Disabled"=w3693) -> ()  [unwired: 2 in, 2 out]
            n2471 = property on="电流步长" class="DigNum (严格)"("Disabled"=w3693) -> ()  [unwired: 2 in, 2 out]
            n2472 = property on="SOC" class="DigNum (严格)"("Disabled"=w3693) -> ()  [unwired: 2 in, 2 out]
            n2473 = property on="充电总安时" class="DigNum (严格)"("Disabled"=w3693) -> ()  [unwired: 2 in, 2 out]
            n2474 = property on="放电总这时" class="DigNum (严格)"("Disabled"=w3693) -> ()  [unwired: 2 in, 2 out]
            n2475 = Not(x=w3700) -> (.not. x?=w3699:bool)
          }
          frame "充放电安时" {
            w3702 = 0
            w3703 = 2
            w3705 = 2
            w3707 = 2
            w3710 = FALSE ("1 6")
            n2476 = property on="电池类型" class="DigNum (严格)"("Disabled"=w3707) -> ()  [unwired: 2 in, 2 out]
            n2477 = property on="电池厂家" class="DigNum (严格)"("Disabled"=w3707) -> ()  [unwired: 2 in, 2 out]
            n2478 = property on="电池地区" class="DigNum (严格)"("Disabled"=w3707) -> ()  [unwired: 2 in, 2 out]
            n2479 = property on="电池组序号" class="DigNum (严格)"("Disabled"=w3707) -> ()  [unwired: 2 in, 2 out]
            n2480 = property on="电池包串联数" class="DigNum (严格)"("Disabled"=w3707) -> ()  [unwired: 2 in, 2 out]
            n2481 = property on="电池包并联数" class="DigNum (严格)"("Disabled"=w3707) -> ()  [unwired: 2 in, 2 out]
            n2482 = property on="电池包安时数" class="DigNum (严格)"("Disabled"=w3707) -> ()  [unwired: 2 in, 2 out]
            n2483 = property on="电池组信息" class="Clust (严格)"("Disabled"=0) -> ()  [unwired: 2 in, 2 out]
            n2484 = property on="车牌号" class="Str"("Disabled"=2) -> ()  [unwired: 2 in, 2 out]
            n2485 = property on="电池包序号" class="DigNum (严格)"("Disabled"=2) -> ()  [unwired: 2 in, 2 out]
            n2486 = property on="充电次数" class="DigNum (严格)"("Disabled"=w3705) -> ()  [unwired: 2 in, 2 out]
            n2487 = property on="充满电时间" class="DigNum (严格)"("Disabled"=w3705) -> ()  [unwired: 2 in, 2 out]
            n2488 = property on="放空时间" class="DigNum (严格)"("Disabled"=w3705) -> ()  [unwired: 2 in, 2 out]
            n2489 = property on="最大允许单体电压" class="DigNum (严格)"("Disabled"=w3703) -> ()  [unwired: 2 in, 2 out]
            n2490 = property on="最大允许总电压" class="DigNum (严格)"("Disabled"=w3703) -> ()  [unwired: 2 in, 2 out]
            n2491 = property on="最大允许温度" class="DigNum (严格)"("Disabled"=w3703) -> ()  [unwired: 2 in, 2 out]
            n2492 = property on="最小允许温度" class="DigNum (严格)"("Disabled"=w3703) -> ()  [unwired: 2 in, 2 out]
            n2493 = property on="最大允许充电电流" class="DigNum (严格)"("Disabled"=w3703) -> ()  [unwired: 2 in, 2 out]
            n2494 = property on="最小允许充电电流" class="DigNum (严格)"("Disabled"=w3703) -> ()  [unwired: 2 in, 2 out]
            n2495 = property on="最小允许单体电压" class="DigNum (严格)"("Disabled"=w3703) -> ()  [unwired: 2 in, 2 out]
            n2496 = property on="电流步长" class="DigNum (严格)"("Disabled"=w3703) -> ()  [unwired: 2 in, 2 out]
            n2497 = property on="SOC" class="DigNum (严格)"("Disabled"=w3703) -> ()  [unwired: 2 in, 2 out]
            n2498 = property on="充电总安时" class="DigNum (严格)"("Disabled"=w3702) -> ()  [unwired: 2 in, 2 out]
            n2499 = property on="放电总这时" class="DigNum (严格)"("Disabled"=w3702) -> ()  [unwired: 2 in, 2 out]
            n2500 = Not(x=w3710) -> (.not. x?=w3709:bool)
          }
          frame "充电次数时间" {
            w3712 = 2
            w3713 = 2
            w3715 = 0
            w3717 = 2
            w3720 = FALSE ("1 6")
            n2501 = property on="电池类型" class="DigNum (严格)"("Disabled"=w3717) -> ()  [unwired: 2 in, 2 out]
            n2502 = property on="电池厂家" class="DigNum (严格)"("Disabled"=w3717) -> ()  [unwired: 2 in, 2 out]
            n2503 = property on="电池地区" class="DigNum (严格)"("Disabled"=w3717) -> ()  [unwired: 2 in, 2 out]
            n2504 = property on="电池组序号" class="DigNum (严格)"("Disabled"=w3717) -> ()  [unwired: 2 in, 2 out]
            n2505 = property on="电池包串联数" class="DigNum (严格)"("Disabled"=w3717) -> ()  [unwired: 2 in, 2 out]
            n2506 = property on="电池包并联数" class="DigNum (严格)"("Disabled"=w3717) -> ()  [unwired: 2 in, 2 out]
            n2507 = property on="电池包安时数" class="DigNum (严格)"("Disabled"=w3717) -> ()  [unwired: 2 in, 2 out]
            n2508 = property on="电池组信息" class="Clust (严格)"("Disabled"=0) -> ()  [unwired: 2 in, 2 out]
            n2509 = property on="车牌号" class="Str"("Disabled"=2) -> ()  [unwired: 2 in, 2 out]
            n2510 = property on="电池包序号" class="DigNum (严格)"("Disabled"=2) -> ()  [unwired: 2 in, 2 out]
            n2511 = property on="充电次数" class="DigNum (严格)"("Disabled"=w3715) -> ()  [unwired: 2 in, 2 out]
            n2512 = property on="充满电时间" class="DigNum (严格)"("Disabled"=w3715) -> ()  [unwired: 2 in, 2 out]
            n2513 = property on="放空时间" class="DigNum (严格)"("Disabled"=w3715) -> ()  [unwired: 2 in, 2 out]
            n2514 = property on="最大允许单体电压" class="DigNum (严格)"("Disabled"=w3713) -> ()  [unwired: 2 in, 2 out]
            n2515 = property on="最大允许总电压" class="DigNum (严格)"("Disabled"=w3713) -> ()  [unwired: 2 in, 2 out]
            n2516 = property on="最大允许温度" class="DigNum (严格)"("Disabled"=w3713) -> ()  [unwired: 2 in, 2 out]
            n2517 = property on="最小允许温度" class="DigNum (严格)"("Disabled"=w3713) -> ()  [unwired: 2 in, 2 out]
            n2518 = property on="最大允许充电电流" class="DigNum (严格)"("Disabled"=w3713) -> ()  [unwired: 2 in, 2 out]
            n2519 = property on="最小允许充电电流" class="DigNum (严格)"("Disabled"=w3713) -> ()  [unwired: 2 in, 2 out]
            n2520 = property on="最小允许单体电压" class="DigNum (严格)"("Disabled"=w3713) -> ()  [unwired: 2 in, 2 out]
            n2521 = property on="电流步长" class="DigNum (严格)"("Disabled"=w3713) -> ()  [unwired: 2 in, 2 out]
            n2522 = property on="SOC" class="DigNum (严格)"("Disabled"=w3713) -> ()  [unwired: 2 in, 2 out]
            n2523 = property on="充电总安时" class="DigNum (严格)"("Disabled"=w3712) -> ()  [unwired: 2 in, 2 out]
            n2524 = property on="放电总这时" class="DigNum (严格)"("Disabled"=w3712) -> ()  [unwired: 2 in, 2 out]
            n2525 = Not(x=w3720) -> (.not. x?=w3719:bool)
          }
          frame "SOC" {
            w3723 = 2
            w3724 = 2
            w3726 = 2
            w3728 = 2
            w3731 = FALSE ("1 6")
            n2526 = property on="电池类型" class="DigNum (严格)"("Disabled"=w3728) -> ()  [unwired: 2 in, 2 out]
            n2527 = property on="电池厂家" class="DigNum (严格)"("Disabled"=w3728) -> ()  [unwired: 2 in, 2 out]
            n2528 = property on="电池地区" class="DigNum (严格)"("Disabled"=w3728) -> ()  [unwired: 2 in, 2 out]
            n2529 = property on="电池组序号" class="DigNum (严格)"("Disabled"=w3728) -> ()  [unwired: 2 in, 2 out]
            n2530 = property on="电池包串联数" class="DigNum (严格)"("Disabled"=w3728) -> ()  [unwired: 2 in, 2 out]
            n2531 = property on="电池包并联数" class="DigNum (严格)"("Disabled"=w3728) -> ()  [unwired: 2 in, 2 out]
            n2532 = property on="电池包安时数" class="DigNum (严格)"("Disabled"=w3728) -> ()  [unwired: 2 in, 2 out]
            n2533 = property on="电池组信息" class="Clust (严格)"("Disabled"=0) -> ()  [unwired: 2 in, 2 out]
            n2534 = property on="车牌号" class="Str"("Disabled"=2) -> ()  [unwired: 2 in, 2 out]
            n2535 = property on="电池包序号" class="DigNum (严格)"("Disabled"=2) -> ()  [unwired: 2 in, 2 out]
            n2536 = property on="充电次数" class="DigNum (严格)"("Disabled"=w3726) -> ()  [unwired: 2 in, 2 out]
            n2537 = property on="充满电时间" class="DigNum (严格)"("Disabled"=w3726) -> ()  [unwired: 2 in, 2 out]
            n2538 = property on="放空时间" class="DigNum (严格)"("Disabled"=w3726) -> ()  [unwired: 2 in, 2 out]
            n2539 = property on="最大允许单体电压" class="DigNum (严格)"("Disabled"=w3724) -> ()  [unwired: 2 in, 2 out]
            n2540 = property on="最大允许总电压" class="DigNum (严格)"("Disabled"=w3724) -> ()  [unwired: 2 in, 2 out]
            n2541 = property on="最大允许温度" class="DigNum (严格)"("Disabled"=w3724) -> ()  [unwired: 2 in, 2 out]
            n2542 = property on="最小允许温度" class="DigNum (严格)"("Disabled"=w3724) -> ()  [unwired: 2 in, 2 out]
            n2543 = property on="最大允许充电电流" class="DigNum (严格)"("Disabled"=w3724) -> ()  [unwired: 2 in, 2 out]
            n2544 = property on="最小允许充电电流" class="DigNum (严格)"("Disabled"=w3724) -> ()  [unwired: 2 in, 2 out]
            n2545 = property on="最小允许单体电压" class="DigNum (严格)"("Disabled"=w3724) -> ()  [unwired: 2 in, 2 out]
